vi "choose a trajectory.vi"(9 "trajectory":i32, 10 "data":waveform(dbl)[](array[waveform]), 11 "bead info":string[](array[string])) -> (2 "trajectory":waveform(dbl) caption="Waveform", 3 "data name":string)   [LabVIEW 2017]
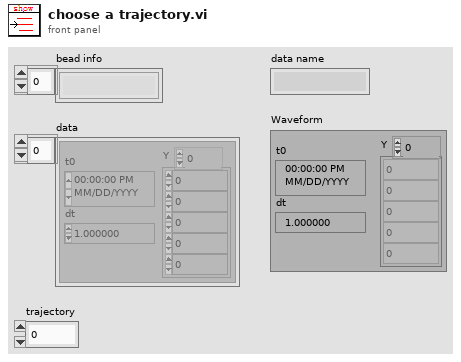
[diagram p1: front panel]
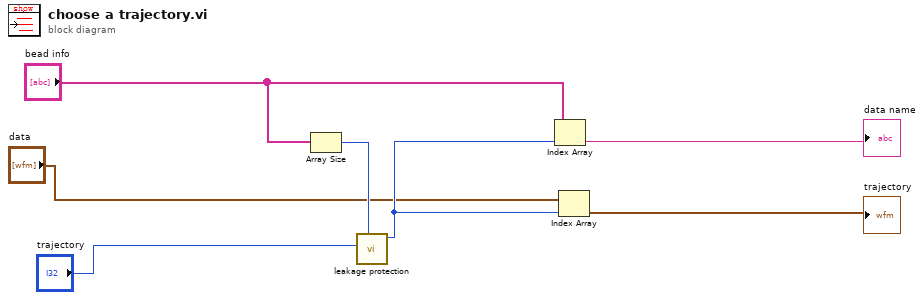
[diagram p0: block diagram]
diagram:
  n1 = Array Size(array="bead info") -> (size(s)=w6:i32)
  n2 = call "leakage protection.vi"("matrix size"=w6, "index in"="trajectory") -> ("index out"=w4:i32)  [unwired: 9 in]
  n3 = Index Array(array="bead info", index=w4) -> (element=→"data name":string)
  n4 = Index Array(array="data", index=w4) -> (element=→"trajectory":waveform(dbl))
